vi "Event Queues Manager_SubVIs-某型振动实验台测试系统.vi"(7 "Mode":T1, 8 "error in":errorcluster, 9 "Front?":bool, 10 "Message":variant, 11 "event":string) -> (0 "error out":errorcluster, 3 "Process1":cluster{"event":string, "Message":variant})   [LabVIEW 2011]
doc: "Use this template to build a VI to use as a subVI."
panel:
  in  "queues":cluster{"Process1":refnum<queue>}
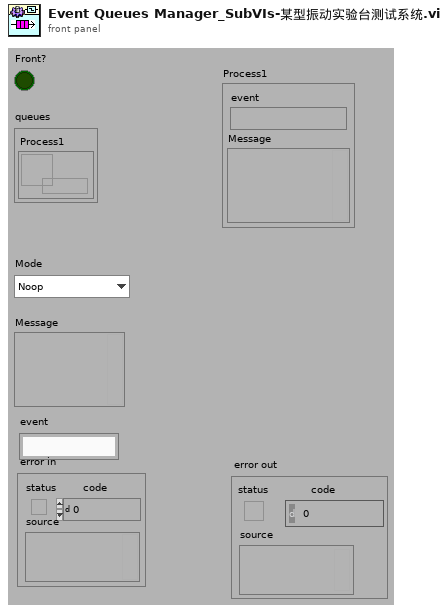
[diagram p1: front panel]
types:
  T1 = typedef "Enum queue_Ctrls-某型振动实验台测试系统.ctl" = enum16{"Noop", "Send Pro1", "Send data", "Get Pro1", "Get data", "Flush Pro1", "Flush data", "Destroy Pro1", "Destroy data"}
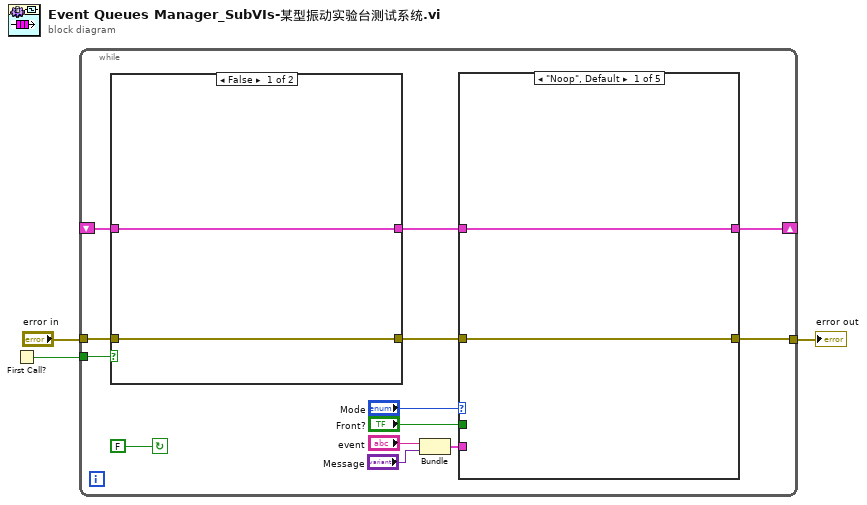
[diagram p0: block diagram]
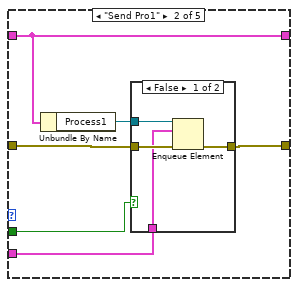
[diagram p2: hidden frame]
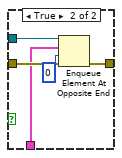
[diagram p3: hidden frame]
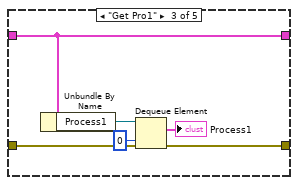
[diagram p4: hidden frame]
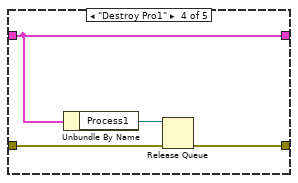
[diagram p5: hidden frame]
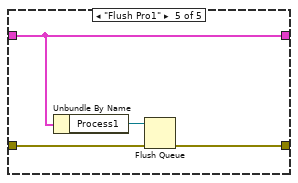
[diagram p6: hidden frame]
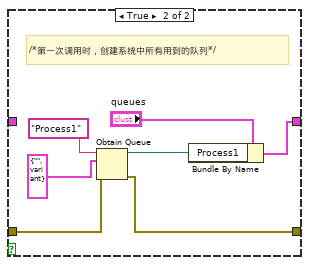
[diagram p7: hidden frame]
diagram:
  n1 = First Call?() -> (First Call?: T/F=w3:bool)
  n2 = while {
    tunnel: w3 -> [w15]
    tunnel: [w11] -> w1
    shift-right: [w10] -> _
    shift-left: _ -> [w9]
    tunnel: "error in" -> [w8]
    stop <- FALSE continue-if-true
    n3 = case shown="False" w15 {
      tunnel: [w49 w54] -> w13
      tunnel: [w48 w51] -> w12
      tunnel: w9 -> [w49 _]
      tunnel: w8 -> [w48 w50]
      frame False {
      }
      frame True {
        # "/*第一次调用时，创建系统中所有用到的队列*/"
        n4 = Obtain Queue(name (unnamed)="Process1", element data type=cluster{"event":string, "Message":variant} {"event"="", "Message"=variant} ("Cluster"), error in (no error)=w50) -> (queue out=w52:refnum<queue>, error out=w51:errorcluster)  [unwired: 2 in, 1 out]
        n5 = Bundle By Name(cluster="queues", "Process1"=w52) -> (w54:cluster{"Process1":refnum<queue>})
      }
    }
    n6 = Bundle("event"="event", "Message"="Message") -> (w5:cluster{"event":string, "Message":variant})  [unwired: 1 out]
    n7 = case shown="\"Noop\", Default" "Mode" {
      tunnel: w13 -> [w18 w22 w36 w40 w46]
      tunnel: w12 -> [w17 w24 w38 w43 w45]
      tunnel: [w17 w23 w37 w42 w44] -> w11
      tunnel: [w18 w22 w36 w40 w46] -> w10
      tunnel: "Front?" -> [_ w21 _ _ _]
      tunnel: w5 -> [_ w19 _ _ _]
      frame "Noop", Default {
      }
      frame "Send Pro1" {
        n8 = Unbundle By Name(w22) -> ("Process1"=w20:refnum<queue>)
        n9 = case shown="False" w21 {
          tunnel: w24 -> [w28 w33]
          tunnel: [w27 w32] -> w23
          tunnel: w20 -> [w26 w30]
          tunnel: w19 -> [w25 w29]
          frame False {
            n10 = Enqueue Element(queue=w26, element=w25, error in (no error)=w28) -> (error out=w27:errorcluster)  [unwired: 3 out]
          }
          frame True {
            n11 = Enqueue Element At Opposite End(queue=w30, element=w29, timeout in ms (-1)=0, error in (no error)=w33) -> (error out=w32:errorcluster)  [unwired: 2 out]
          }
        }
      }
      frame "Get Pro1" {
        n12 = Unbundle By Name(w36) -> ("Process1"=w39:refnum<queue>)
        n13 = Dequeue Element(queue=w39, timeout in ms (-1)=0, error in (no error)=w38) -> (element=→"Process1":cluster{"event":string, "Message":variant}, error out=w37:errorcluster)  [unwired: 2 out]
      }
      frame "Destroy Pro1" {
        n14 = Unbundle By Name(w40) -> ("Process1"=w41:refnum<queue>)
        n15 = Release Queue(queue=w41, error in (no error)=w43) -> (error out=w42:errorcluster)  [unwired: 3 out]
      }
      frame "Flush Pro1" {
        n16 = Unbundle By Name(w46) -> ("Process1"=w47:refnum<queue>)
        n17 = Flush Queue(queue=w47, error in (no error)=w45) -> (error out=w44:errorcluster)  [unwired: 2 out]
      }
    }
  }
  "error out" <- w1
